vi "Initialize.vi"(8 "error in (no error)":errorcluster, 10 "General Settings":T1, 11 "IPC_Communication in":refnum<class "IP_Communication.lvclass">) -> (0 "error out":errorcluster, 3 "IPC_Communication out":refnum<class "IP_Communication.lvclass">)   [LabVIEW 2020, in "Communication Classes.lvlib" / "IP_Communication.lvclass"]
uses:
  IP_Communication.lvclass
  typedefs/General Settings.ctl
  typedefs/Endpoint Tag.ctl
  IP_Communication.lvclass/IP_Communication.ctl
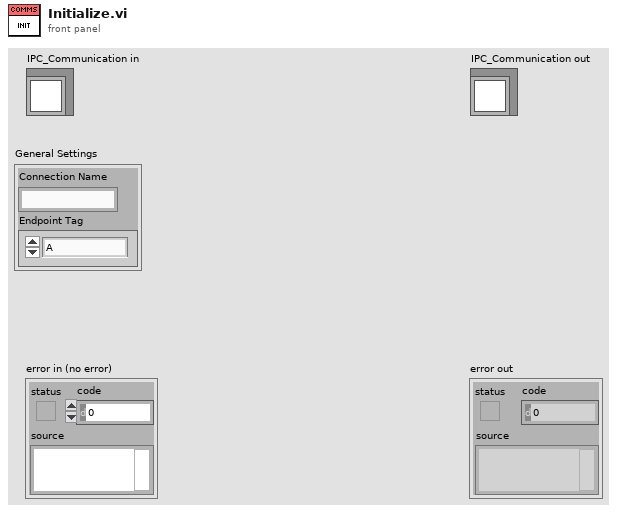
[diagram p1: front panel]
types:
  T1 = typedef "Communication Classes.lvlib/IP_Communication.lvclass/General Settings.ctl" = cluster{"Connection Name":string, "Endpoint Tag":T2}
  T2 = typedef "Communication Classes.lvlib/IP_Communication.lvclass/Endpoint Tag.ctl" = enum8{"A", "B"}
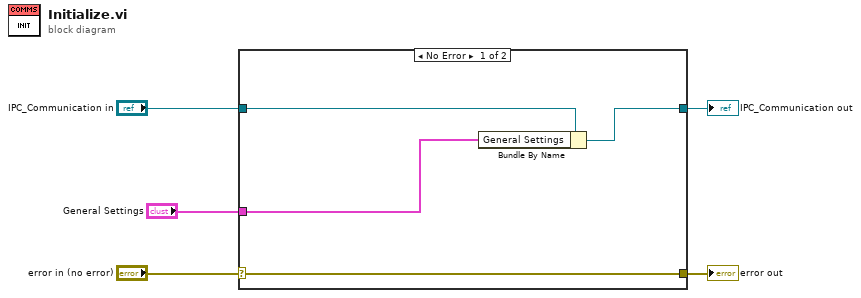
[diagram p0: block diagram]
diagram:
  n1 = case shown="No Error" "error in (no error)" {
    selector: "error in (no error)" -> [w9 w11]
    tunnel: [w9 w11] -> w4
    tunnel: [w6 w10] -> w2
    tunnel: "IPC_Communication in" -> [w8 w10]
    tunnel: "General Settings" -> [w7 _]
    frame No Error {
      n2 = Bundle By Name(cluster=w8, "General Settings"=w7) -> (w6:refnum<class "IP_Communication.lvclass">)
    }
    frame Error {
    }
  }
  "error out" <- w4
  "IPC_Communication out" <- w2
